vi "server.vi"() -> ()   [LabVIEW 2017]
uses:
  1-webservice/data.vi
  <vilib>/Waveform/WDTOps.llb/WDT Append Waveforms DBL.vi
panel:
  out "data":dbl
  out "Numeric":dbl
  in  "stop 2":bool
  out "bytes written":i32
  out "bytes sent":i32
  in  "stop":bool
  out "Waveform Chart":waveform(dbl)(graph)
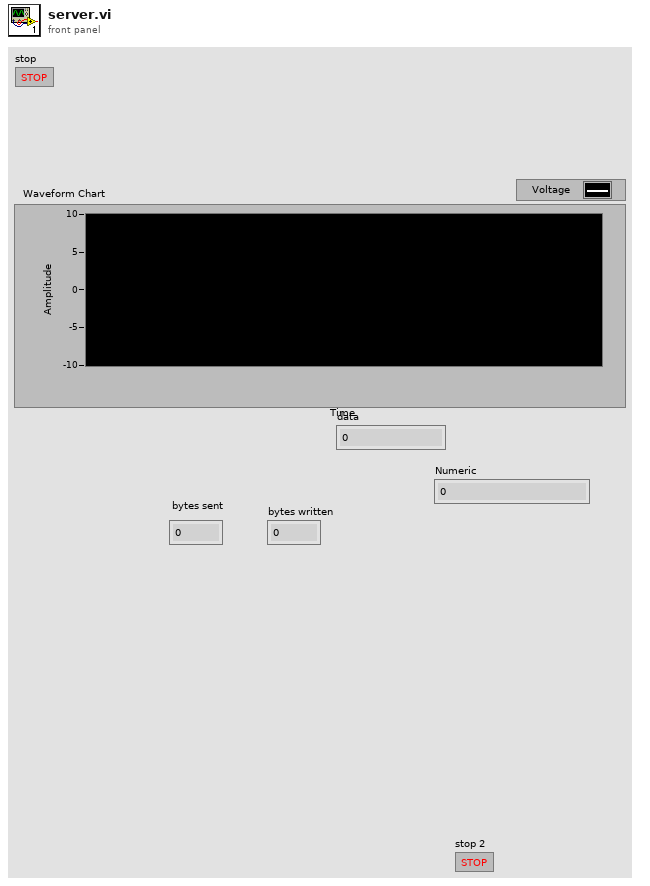
[diagram p1: front panel]
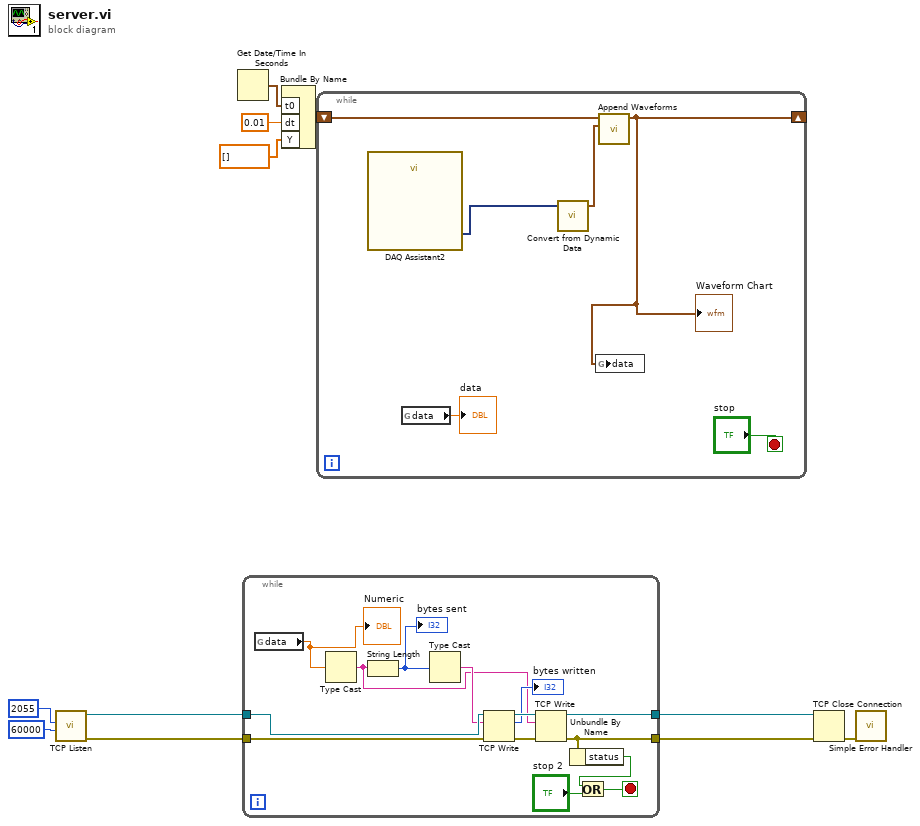
[diagram p0: block diagram]
diagram:
  n1 = call <vilib>:"TCP Listen.vi"("timeout ms (wait forever: -1)"=60000, "port"=u16 2055) -> ("error out"=w4:errorcluster, "connection ID"=w5:refnum<k5>)  [unwired: 5 in, 3 out]
  n2 = Get Date/Time In Seconds() -> (seconds since 1Jan1904=w9:timestamp)
  n3 = while {
    tunnel: w5 -> [w24]
    tunnel: w4 -> [w23]
    tunnel: [w19] -> w3
    tunnel: [w15] -> w2
    stop <- w17 stop-if-true
    n4 = global read "data.vi" "data"() -> (w12:dbl)
    "Numeric" <- w12
    n5 = Type Cast(x=w12) -> (*(type *) &x=w13:string)  [unwired: 1 out]
    n6 = String Length(string=w13) -> (length=w25:i32)
    "bytes sent" <- w25
    n7 = Type Cast(x=w25) -> (*(type *) &x=w22:string)  [unwired: 1 out]
    n8 = TCP Write(connection ID=w24, data in=w22, error in (no error)=w23) -> (connection ID out=w21:refnum<k5>, bytes written=→"bytes written":i32, error out=w20:errorcluster)  [unwired: 1 out]
    n9 = TCP Write(connection ID=w21, data in=w13, error in (no error)=w20) -> (connection ID out=w19:refnum<k5>, error out=w15:errorcluster)  [unwired: 2 out]
    n10 = Unbundle By Name(w15) -> ("status"=w14:bool)
    n11 = Or(x=w14, y="stop 2") -> (x .or. y?=w17:bool)
  }
  n12 = Bundle By Name("t0"=w9, "dt"=0.01, "Y"=dbl[] []) -> (w8:waveform(dbl))  [unwired: 1 in]
  n13 = while {
    shift-right: [w28] -> _
    shift-left: w8 -> [w31]
    stop <- "stop" stop-if-true
    n14 = call "DAQ Assistant2"() -> ("data"=w27:dynamicdata)  [unwired: 17 in, 2 out]
    n15 = global read "data.vi" "data"() -> (→"data":dbl)
    n16 = call "Convert from Dynamic Data"("Dynamic Data Type"=w27) -> ("Waveform"=w30:waveform(dbl))  [unwired: 3 in]
    n17 = call-poly <vilib>:"Append Waveforms.vi"("waveform B"=w30, "waveform A"=w31) -> ("waveform out"=w28:waveform(dbl))  [unwired: 8 in, 1 out]
    "Waveform Chart" <- w28
    n18 = global write "data.vi" "data"(w28) -> ()
  }
  n19 = TCP Close Connection(connection ID=w3, error in (no error)=w2) -> (error out=w1:errorcluster)  [unwired: 1 in, 1 out]
  n20 = call <vilib>:"Simple Error Handler.vi"("error in (no error)"=w1) -> ()  [unwired: 4 in, 5 out]
